vi "sub_conv_map_gen_v2.vi"(11 "code type":T1(ring)) -> (1 "output in decimal":u32[][](array[numeric]), 3 "state transition":u32[][](array[numeric]))   [LabVIEW 2014]
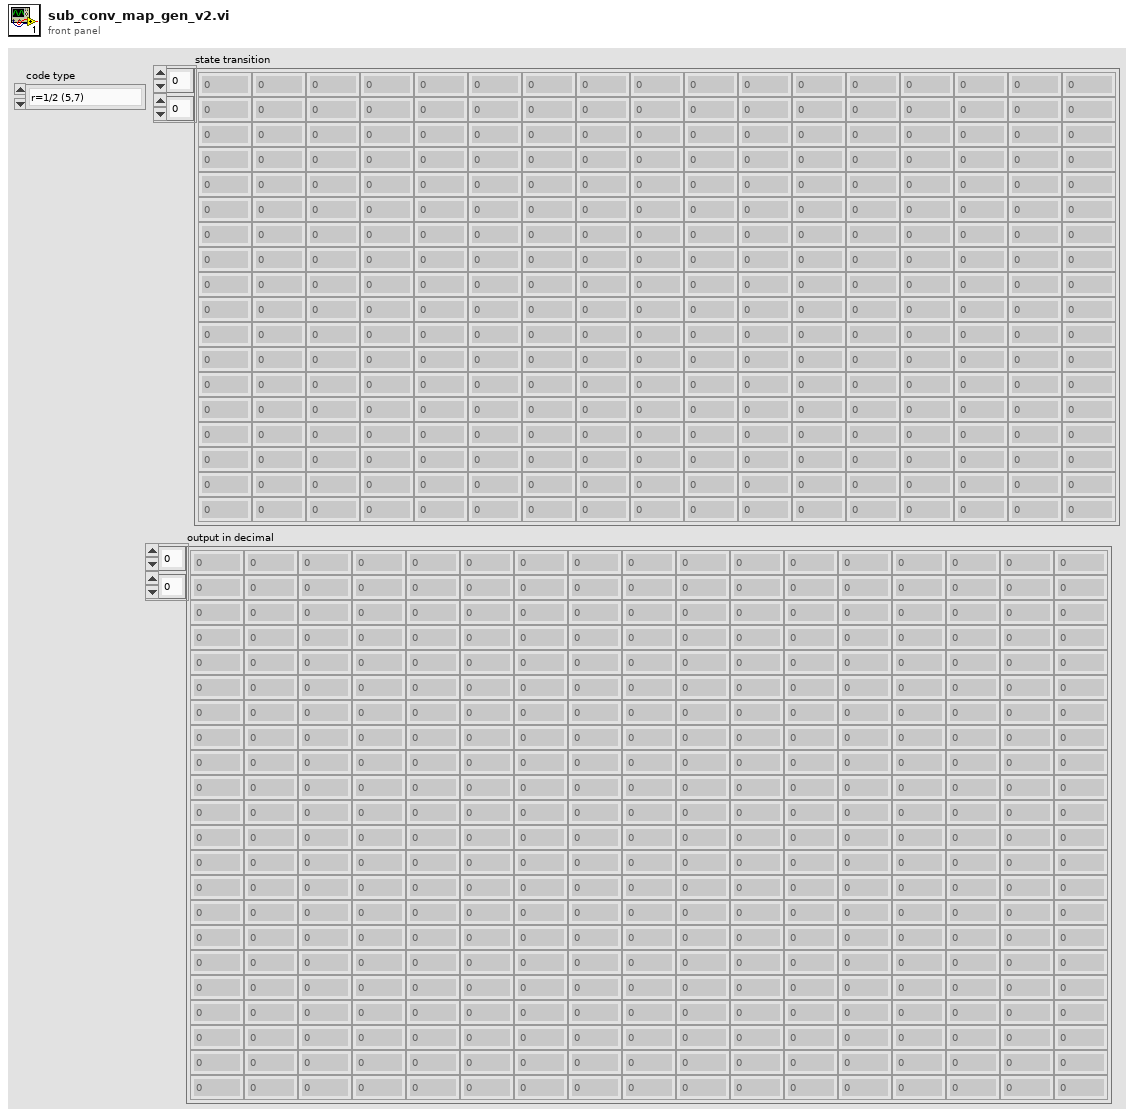
[diagram p1: front panel]
types:
  T1 = enum16{"r=1/2 (5,7)", "r=1/2 (13,17)", "r=1/4 (25,27,33,37)"}
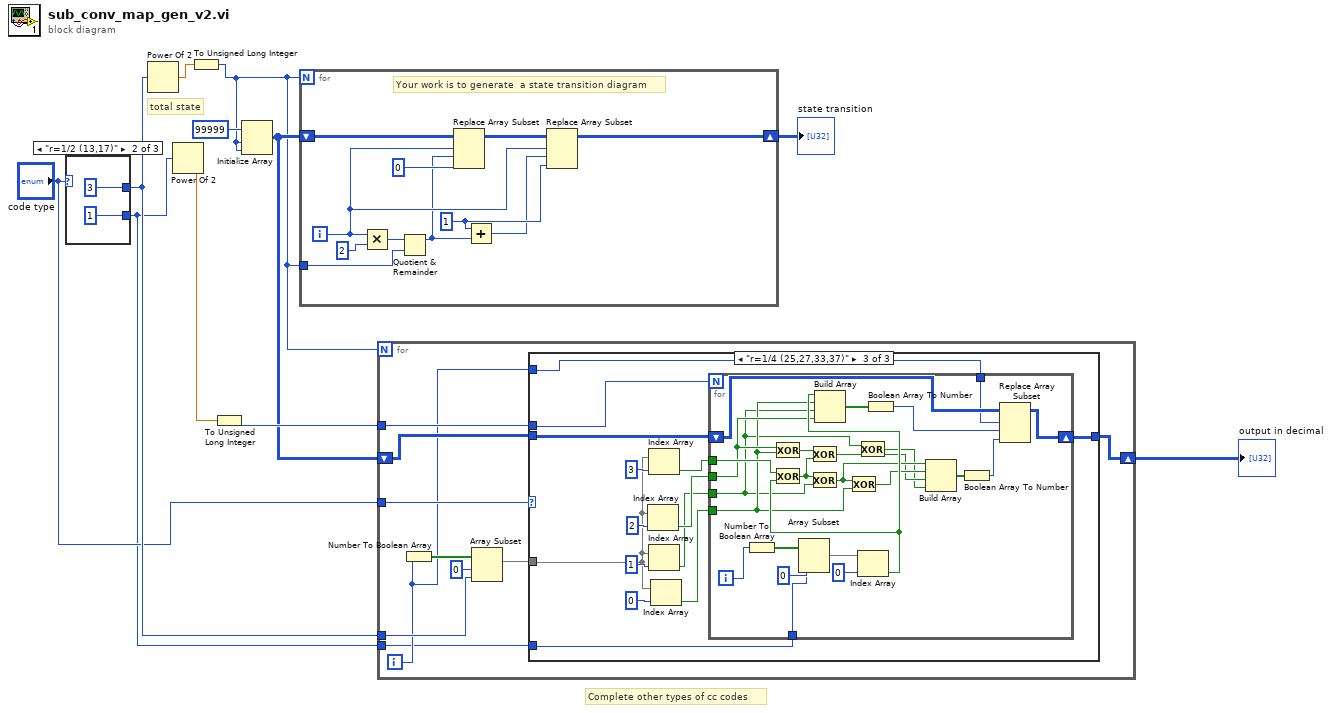
[diagram p0: block diagram]
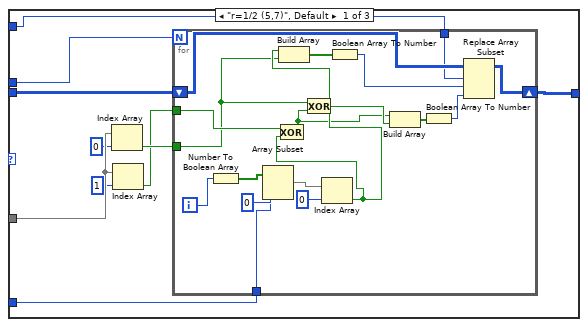
[diagram p2: hidden frame]
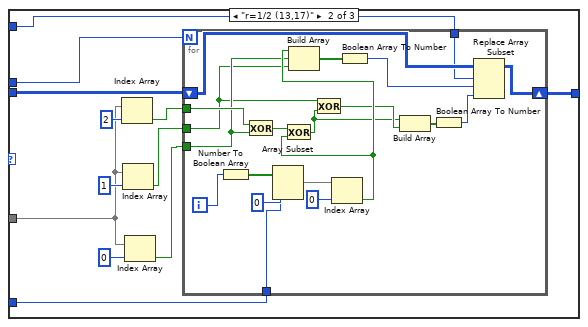
[diagram p3: hidden frame]
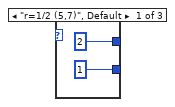
[diagram p4: hidden frame]
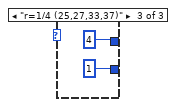
[diagram p5: hidden frame]
diagram:
  # "Complete other types of cc codes"
  # "total state"
  n1 = case shown="\"r=1/2 (13,17)\"" "code type" {
    tunnel: [u32 2 u32 3 u32 4] -> w9
    tunnel: [u32 1 u32 1 u32 1] -> w2
    frame "r=1/2 (5,7)", Default {
    }
    frame "r=1/2 (13,17)" {
    }
    frame "r=1/4 (25,27,33,37)" {
    }
  }
  n2 = Power Of 2(x=w9) -> (2^x=w7:dbl)
  n3 = Power Of 2(x=w2) -> (2^x=w6:dbl)
  n4 = To Unsigned Long Integer(number=w7) -> (unsigned 32bit integer=w1:u32)
  n5 = To Unsigned Long Integer(number=w6) -> (unsigned 32bit integer=w5:u32)
  n6 = Initialize Array(u32 99999, w1, w1) -> (w4:u32[][])
  n7 = for {
    N: w1 -> [_]
    shift-right: [w18] -> w10
    shift-left: w4 -> [w28]
    tunnel: w1 -> [w25]
    i -> [w22]
    w20 = u32 1
    # "Your work is to generate  a state transition diagram"
    n8 = Multiply(x=w22, y=u32 2) -> (x*y=w26:u32)
    n9 = Quotient & Remainder(x=w26, y=w25) -> (x-y*floor(x/y)=w21:u32)  [unwired: 1 out]
    n10 = Replace Array Subset(array=w28, new element=u32 0, index (row)=w22, index (col)=w21) -> (w23:u32[][])
    n11 = Add(x=w20, y=w21) -> (x+y=w19:u32)
    n12 = Replace Array Subset(array=w23, new element=w20, index (row)=w22, index (col)=w19) -> (w18:u32[][])
  }
  "state transition" <- w10
  n13 = for {
    N: w1 -> [_]
    tunnel: w5 -> [w38]
    tunnel: w2 -> [w30]
    tunnel: w9 -> [w36]
    tunnel: "code type" -> [w34]
    shift-right: [w32] -> w3
    shift-left: w4 -> [w33]
    i -> [w31]
    n14 = Number To Boolean Array(number=w31) -> (Boolean array=w37:bool[])
    n15 = Array Subset(array=w37, index=0, length=w36) -> (w35:bool[])
    n16 = case shown="\"r=1/4 (25,27,33,37)\"" w34 {
      tunnel: w38 -> [w48 w75 w104]
      tunnel: w30 -> [w47 w73 w106]
      tunnel: w35 -> [w46 w71 w100]
      tunnel: [w39 w72 w102] -> w32
      tunnel: w33 -> [w41 w74 w105]
      tunnel: w31 -> [w40 w76 w103]
      frame "r=1/2 (5,7)", Default {
        n17 = Index Array(array=w46, index=0) -> (element=w43:bool)
        n18 = Index Array(array=w46, index=1) -> (element=w42:bool)
        n19 = for {
          N: w48 -> [_]
          tunnel: w47 -> [w63]
          tunnel: w42 -> [w52]
          tunnel: w43 -> [w51]
          shift-right: [w54] -> w39
          shift-left: w41 -> [w58]
          tunnel: w40 -> [w56]
          i -> [w66]
          n20 = Number To Boolean Array(number=w66) -> (Boolean array=w65:bool[])
          n21 = Array Subset(array=w65, index=0, length=w63) -> (w62:bool[])
          n22 = Index Array(array=w62, index=0) -> (element=w53:bool)
          n23 = Exclusive Or(1:w53, 2:w52) -> (0:w49:bool)
          n24 = Build Array(w53, w51) -> (w59:bool[])
          n25 = Exclusive Or(1:w49, 2:w51) -> (0:w50:bool)
          n26 = Boolean Array To Number(Boolean array=w59) -> (number=w55:u32)
          n27 = Build Array(w49, w50) -> (w60:bool[])
          n28 = Boolean Array To Number(Boolean array=w60) -> (number=w57:u32)
          n29 = Replace Array Subset(array=w58, new element=w57, index (row)=w56, index (col)=w55) -> (w54:u32[][])
        }
      }
      frame "r=1/2 (13,17)" {
        n30 = Index Array(array=w71, index=2) -> (element=w69:bool)
        n31 = Index Array(array=w71, index=1) -> (element=w68:bool)
        n32 = Index Array(array=w71, index=0) -> (element=w67:bool)
        n33 = for {
          N: w75 -> [_]
          tunnel: w73 -> [w95]
          tunnel: w68 -> [w79]
          tunnel: w67 -> [w81]
          shift-right: [w86] -> w72
          shift-left: w74 -> [w90]
          tunnel: w76 -> [w88]
          tunnel: w69 -> [w82]
          i -> [w98]
          n34 = Number To Boolean Array(number=w98) -> (Boolean array=w97:bool[])
          n35 = Exclusive Or(1:w81, 2:w82) -> (0:w80:bool)
          n36 = Array Subset(array=w97, index=0, length=w95) -> (w94:bool[])
          n37 = Index Array(array=w94, index=0) -> (element=w85:bool)
          n38 = Exclusive Or(1:w85, 2:w80) -> (0:w83:bool)
          n39 = Build Array(w85, w81, w79) -> (w91:bool[])
          n40 = Exclusive Or(1:w83, 2:w79) -> (0:w84:bool)
          n41 = Boolean Array To Number(Boolean array=w91) -> (number=w87:u32)
          n42 = Build Array(w83, w84) -> (w92:bool[])
          n43 = Boolean Array To Number(Boolean array=w92) -> (number=w89:u32)
          n44 = Replace Array Subset(array=w90, new element=w89, index (row)=w88, index (col)=w87) -> (w86:u32[][])
        }
      }
      frame "r=1/4 (25,27,33,37)" {
        n45 = Index Array(array=w100, index=2) -> (element=w109:bool)
        n46 = Index Array(array=w100, index=3) -> (element=w99:bool)
        n47 = Index Array(array=w100, index=1) -> (element=w108:bool)
        n48 = Index Array(array=w100, index=0) -> (element=w107:bool)
        n49 = for {
          N: w104 -> [_]
          tunnel: w106 -> [w133]
          tunnel: w108 -> [w114]
          tunnel: w107 -> [w117]
          shift-right: [w124] -> w102
          shift-left: w105 -> [w128]
          tunnel: w103 -> [w126]
          tunnel: w109 -> [w121]
          tunnel: w99 -> [w122]
          i -> [w136]
          n50 = Number To Boolean Array(number=w136) -> (Boolean array=w135:bool[])
          n51 = Exclusive Or(1:w117, 2:w121) -> (0:w120:bool)
          n52 = Array Subset(array=w135, index=0, length=w133) -> (w132:bool[])
          n53 = Index Array(array=w132, index=0) -> (element=w123:bool)
          n54 = Exclusive Or(1:w123, 2:w122) -> (0:w119:bool)
          n55 = Exclusive Or(1:w119, 2:w120) -> (0:w115:bool)
          n56 = Exclusive Or(1:w114, 2:w119) -> (0:w118:bool)
          n57 = Build Array(w123, w117, w114, w121) -> (w129:bool[])
          n58 = Exclusive Or(1:w117, 2:w118) -> (0:w116:bool)
          n59 = Exclusive Or(1:w115, 2:w114) -> (0:w113:bool)
          n60 = Boolean Array To Number(Boolean array=w129) -> (number=w125:u32)
          n61 = Build Array(w118, w116, w115, w113) -> (w130:bool[])
          n62 = Boolean Array To Number(Boolean array=w130) -> (number=w127:u32)
          n63 = Replace Array Subset(array=w128, new element=w127, index (row)=w126, index (col)=w125) -> (w124:u32[][])
        }
      }
    }
  }
  "output in decimal" <- w3
